vi "Convert from DataGrid String.vi"(10 "Display Style":T1, 11 "DataGrid String in":string) -> (3 "Popup String out":string)   [LabVIEW 2018, in "String Data Type.lvclass"]
uses:
  String Data Type.lvclass
  Display Style Enum.ctl
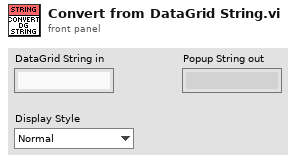
[diagram p1: front panel]
types:
  T1 = typedef "String Data Type.lvclass/Display Style Enum.ctl" = enum16{"Normal", "'\\' Codes", "Hex"}
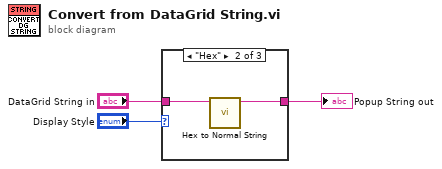
[diagram p0: block diagram]
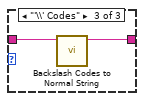
[diagram p3: hidden frame]
diagram:
  n1 = case shown="\"Hex\"" "Display Style" {
    tunnel: "DataGrid String in" -> [w4 w6 w8]
    tunnel: [w4 w5 w7] -> w1
    frame "Normal" {
    }
    frame "Hex" {
      n2 = call "Hex to Normal String.vi"("Hex String in"=w6) -> ("Normal String out"=w5:string)  [unwired: 10 in]
    }
    frame "'\\' Codes" {
      n3 = call "Backslash Codes to Normal String.vi"("Backslash String in"=w8) -> ("Normal String out"=w7:string)  [unwired: 10 in]
    }
  }
  "Popup String out" <- w1
